vi "DecodeData.vi"(10 "data":u8[](array[numeric]), 11 "dataType":string) -> (3 "eu data out":dbl[](array[numeric]))   [LabVIEW 2019, in "HLA Custom Device Engine.lvlib"]
uses:
  HLA Custom Device Engine.lvlib
  Data Encoding_Decoding/HLA Data Conversion.lvlib
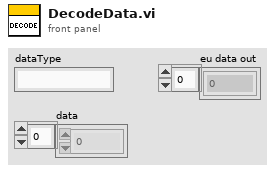
[diagram p1: front panel]
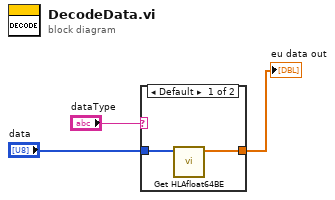
[diagram p0: block diagram]
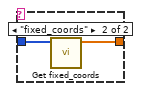
[diagram p2: hidden frame]
diagram:
  n1 = case shown="Default" "dataType" {
    tunnel: [w5 w7] -> w1
    tunnel: "data" -> [w4 w6]
    frame Default {
      n2 = call "Get HLAfloat64BE.vi"("raw data in"=w4) -> ("eu data out"=w5:dbl[])  [unwired: 9 in, 1 out]
    }
    frame "fixed_coords" {
      n3 = call "Get fixed_coords.vi"("raw data in"=w6) -> ("eu data out"=w7:dbl[])  [unwired: 9 in, 1 out]
    }
  }
  "eu data out" <- w1
